vi "20211001_01.vi"() -> ()   [LabVIEW 2019]
panel:
  out "XOR":bool
  in  "Y":bool
  in  "X":bool
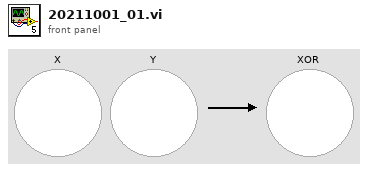
[diagram p1: front panel]
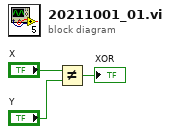
[diagram p0: block diagram]
diagram:
  n1 = Not Equal?(x="X", y="Y") -> (x != y?=→"XOR":bool)
